vi "SG.vi"() -> ()   [LabVIEW 2014]
uses:
  <vilib>/Simulation/Scripting/Companion Diagram/SimConfigNode/SimParams.ctl
  <vilib>/Simulation/Scripting/Companion Diagram/SimConfigNode/_simSolvers.ctl
  <vilib>/Simulation/Implementation/Shared/SIMSCR Execution Mode.ctl
  <vilib>/Simulation/Param Hierarchy/Typedefs/SIMPH Param Control Actions.ctl
  <vilib>/Simulation/Implementation/Shared/SIM limit type.ctl
  <vilib>/Simulation/Implementation/Shared/NILVSim_ParamChanged.vi
  <vilib>/Simulation/Implementation/Shared/NILVSIM_BeginStep.vi
  <vilib>/Simulation/DataSources/Implementation/NILVSim Step.llb/SIM Step (scalar).vi
  <vilib>/Simulation/ContinuousLinear/Implementation/NILVSim Transport Delay.llb/SIM Transport Delay Distributor (scalar).vi
  <vilib>/Simulation/ContinuousLinear/Implementation/NILVSim Integrator new.llb/SIM Integrator distributor (scalar).vi
  <vilib>/Simulation/ContinuousLinear/Implementation/NILVSim Transport Delay.llb/SIM Transport Delay Collector (scalar).vi
  <vilib>/Simulation/SignalDisplay/Implementation/NILVSim Time Waveform.llb/SIM Time Waveform (scalar).vi
  <vilib>/Simulation/ContinuousLinear/Implementation/NILVSim Integrator new.llb/SIM Integrator collector (scalar).vi
  <vilib>/Simulation/Implementation/Shared/NILVSim_Manager.vi
  <vilib>/Utility/error.llb/Clear Errors.vi
  <vilib>/Simulation/Implementation/Shared/NILVSim_FinalizeModel.vi
  <vilib>/Simulation/Implementation/Shared/SIM Unbundle Sim Info.vi
  <vilib>/Simulation/Implementation/Shared/NILVSim_Initialize.vi
  <vilib>/Simulation/Utility/Implementation/NILVSim Get Time and IsAcceptedStep.vi
  <vilib>/Simulation/Implementation/Shared/SIMSH Read Queue.vi
  <vilib>/Simulation/Implementation/Shared/NILVSim_GetModelError.vi
  <vilib>/Simulation/Implementation/Shared/SIM Bundle Sim Info.vi
  <vilib>/Simulation/Scripting/Companion Diagram/SimConfigNode/SimDog.xnode
  <vilib>/Simulation/Implementation/XNodeFramework/SimXNode/SimX.xnode
  <vilib>/Simulation/ContinuousLinear/Implementation/NILVSim Integrator new.llb/SIM Integrator (scalar).vi
  <vilib>/Simulation/ContinuousLinear/Implementation/NILVSim Transport Delay.llb/SIM Transport Delay Indirect (scalar).vi
  <vilib>/Simulation/Implementation/Shared/NI_SIM_Implementation.lvlib
panel:
  in  "Ku":dbl=1.21
  in  "Flujo inicial en tuberia":dbl=2.0
  out "Altura":waveform(dbl)(graph)
  in  "H0":dbl=2.0
  in  "F1":dbl=2.0
  out "Perturbacion":dbl caption="ISE 2"
  in  "Amplitud perturbacion":dbl=0.1
  out "Tank Control ZN C.L.":dbl(slide) scale=0.0..2.0
  in  "K1":dbl=1.21
  in  "A1":dbl=2.0
  # "Identificación depósito"
  # "Flujo de entrada"
  # "PERTURBACIÓN"
  # "SISTEMA"
  # "CONTROLADOR ZN C.L."
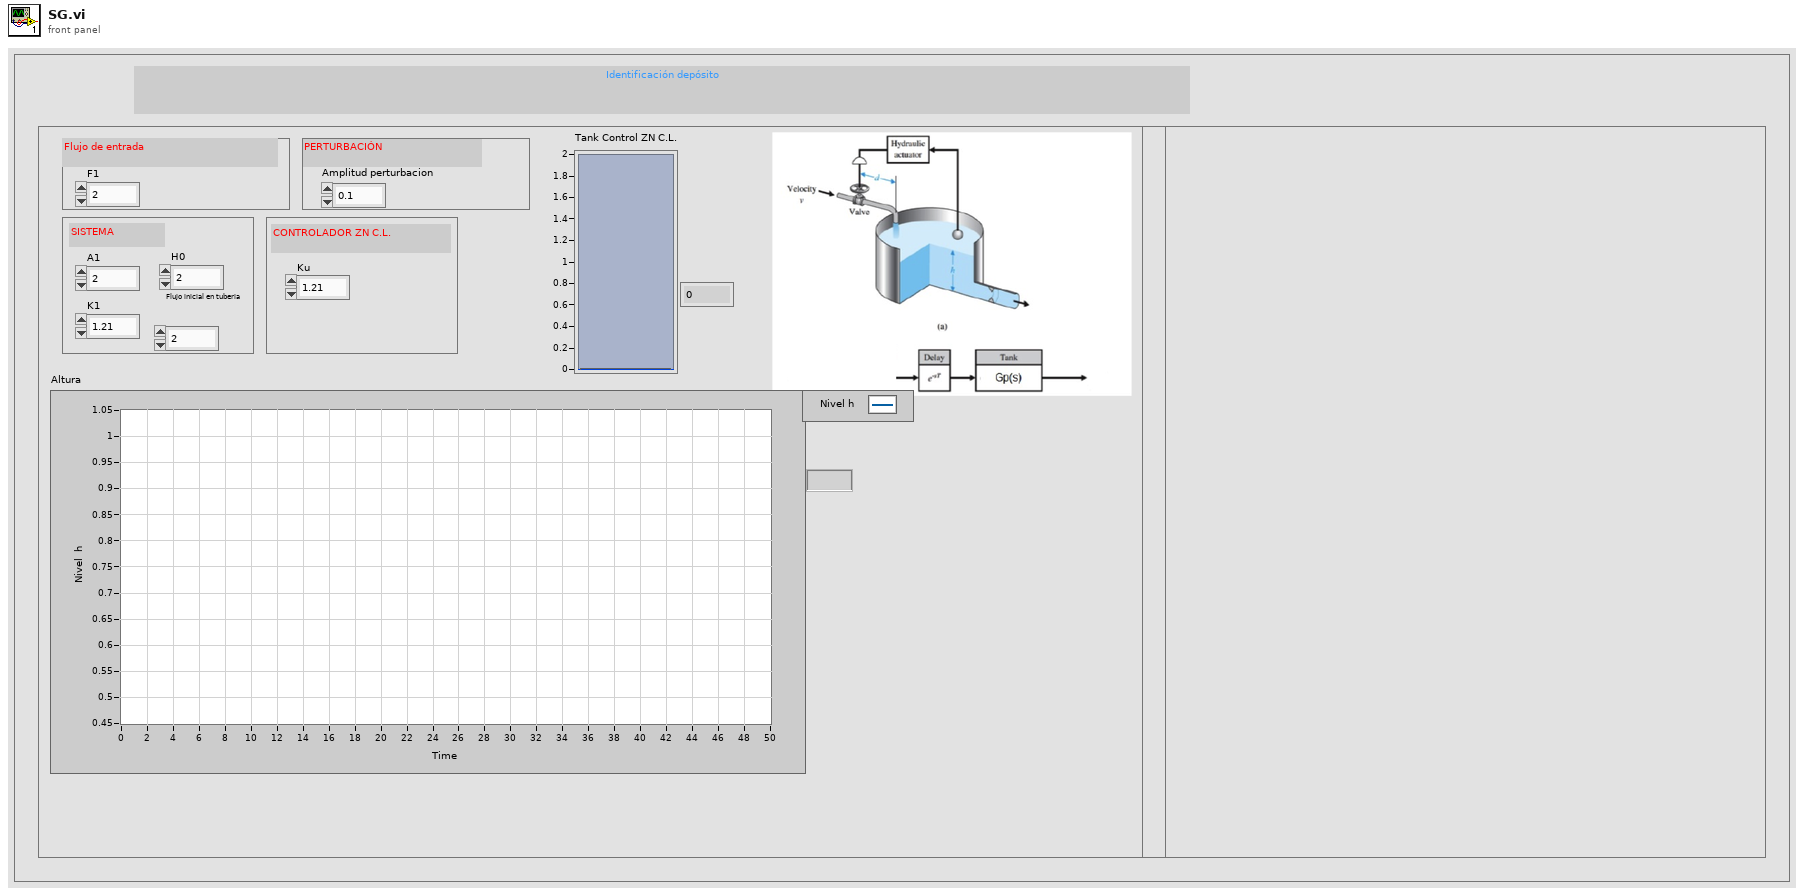
[diagram p1: front panel]
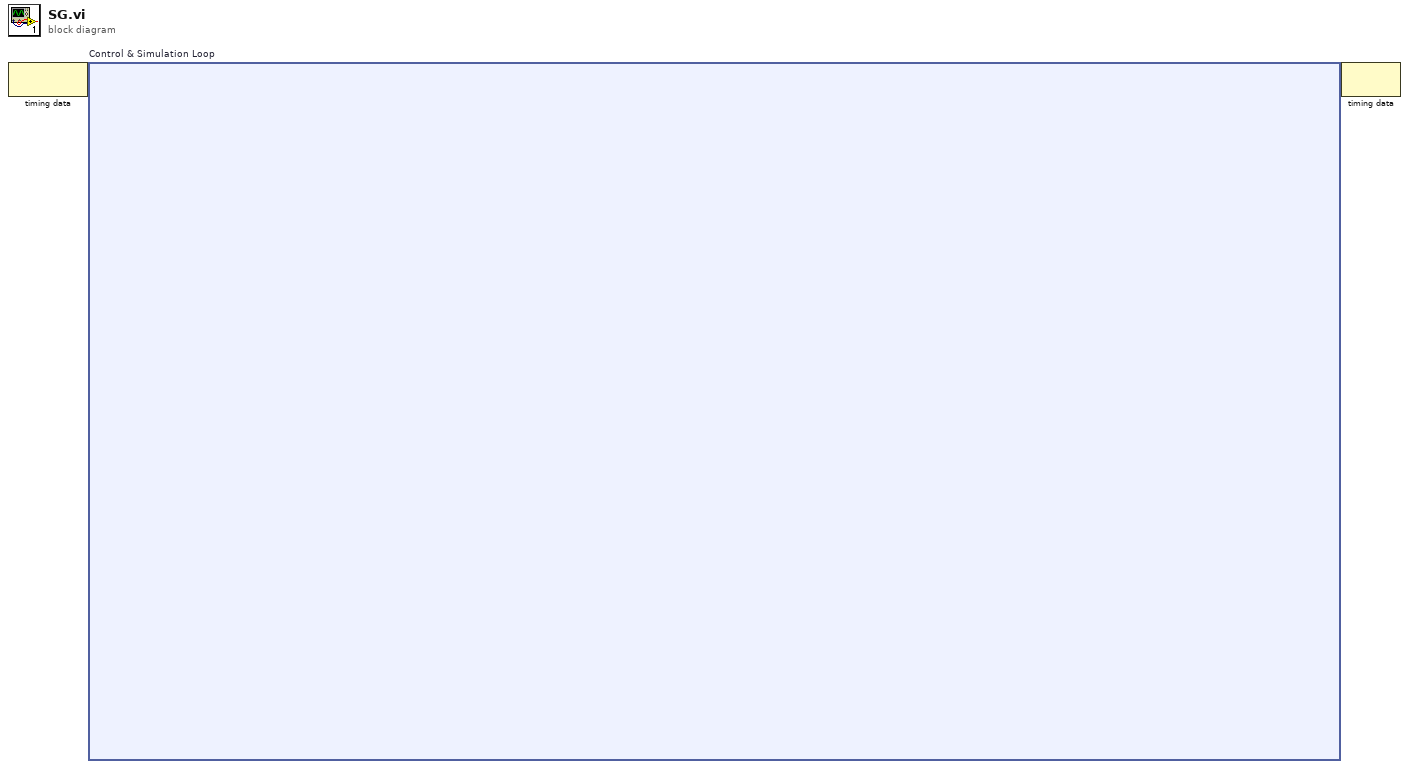
[diagram p0: block diagram]
diagram:
  n1 = node-c288() -> (w2:variant)  [unwired: 1 in]
  n2 = node-c254 "Control & Simulation Loop"(w2) -> (w1:variant)
  n3 = node-c288(w1) -> ()  [unwired: 1 out]
